vi "Built Betweed and.vi"(7 "Where/And":string(combo)="and", 8 "error in (no error)":errorcluster, 9 "End DateTime":string, 10 "Start DateTime":string, 11 "Column Name":string) -> (0 "error out":errorcluster, 3 "Between DateTime":string)   [LabVIEW 2021, in "DataBase_SQL.lvclass"]
uses:
  <userlib>/John_Lib/DataBase/DataBase_SQL/DataBase_SQL.lvclass
  <userlib>/John_Lib/DataBase/DataBase_SQL/DataBase_SQL.lvclass/DataBase_SQL.ctl
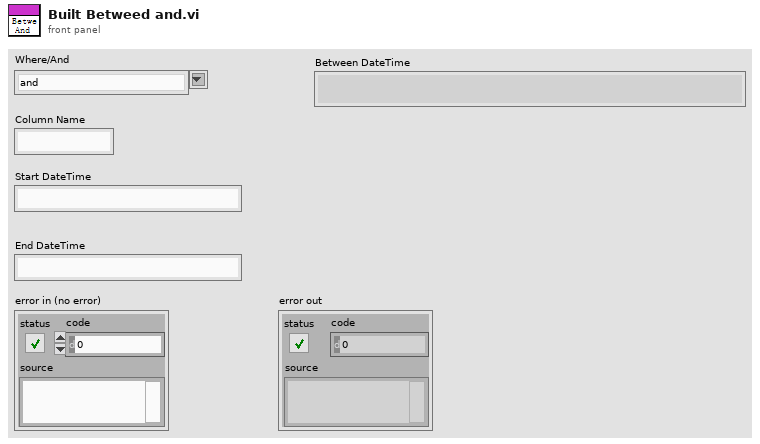
[diagram p1: front panel]
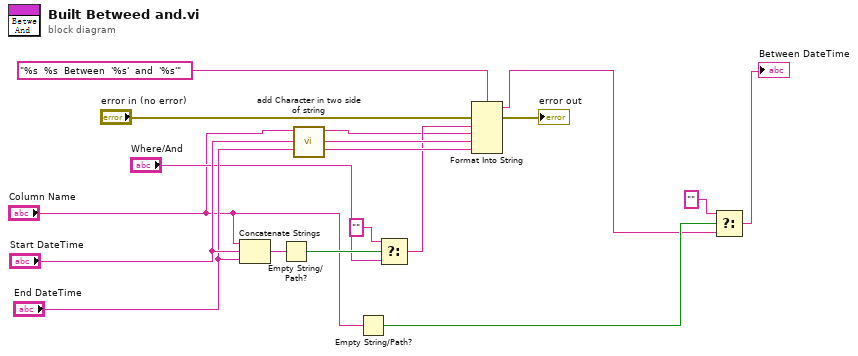
[diagram p0: block diagram]
diagram:
  n1 = Concatenate Strings("Column Name", "Start DateTime", "End DateTime") -> (w11:string)
  n2 = Empty String/Path?(string/path=w11) -> (empty?=w10:bool)
  n3 = call <userlib>:"add Character in two side of string.vi"("Sting In"="Column Name") -> ("String Out"=w1:string)  [unwired: 10 in]
  n4 = Empty String/Path?(string/path="Column Name") -> (empty?=w5:bool)
  n5 = Select(t="", s=w10, f="Where/And") -> (s? t:f=w7:string)
  n6 = Format Into String(format string="%s  %s  Between  '%s'  and  '%s'", error in="error in (no error)", w7, w1, "Start DateTime", "End DateTime") -> (resulting string=w4:string, error out=→"error out":errorcluster)  [unwired: 1 in]
  n7 = Select(t="", s=w5, f=w4) -> (s? t:f=→"Between DateTime":string)
